vi "Complex Inverse Matrix (Cholesky).vi"(3 "Input Matrix":T1) -> (0 "error":i32, 1 "Inverse Matrix":T1)   [LabVIEW 2014, in "NI_AALBase.lvlib"]
doc: "Finds the <B>Inverse Matrix</B>, if it exists, of the <B>Input Matrix</B>, using Cholesky factorization."
uses:
  NI_AALBase.lvlib
  ComplexMatrix.ctl
  lvanlys.dll
  NI_Matrix.lvlib
panel:
  # "Complex Inverse Matrix (Cholesky)"
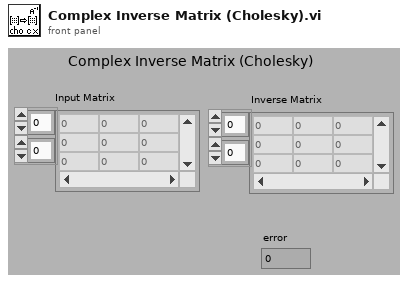
[diagram p1: front panel]
types:
  T1 = typedef "NI_Matrix.lvlib/ComplexMatrix.ctl" = cdb[][]
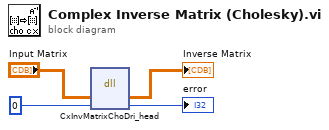
[diagram p0: block diagram]
diagram:
  n1 = dll-call lib="C:/Program Files (x86)/National Instruments/LabVIEW 2014/resource/lvanlys.*" fn="CxInvMatrixChoDri_head"("Input Matrix"="Input Matrix", "error"=0) -> ("Input Matrix"=→"Inverse Matrix":T1, "error"=→"error":i32)  [unwired: 4 in, 2 out]
